vi "Aurora Reader (Dual Port).vi"(2 "aurora rx dual reference":T1, 12 "ready for output":bool=TRUE) -> (4 "data":bool[](array[boolean]), 10 "output valid":bool)   [LabVIEW 2019]
uses:
  <vilib>/eio/EIONode/EIONode.xnode
  <instrlib>/_niInstr/Data Formatting/v1/FPGA/niInstr Data Formatting v1 FPGA.lvlib
  <instrlib>/_niInstr/Data Formatting/v1/FPGA/Private/Convert/U64 array to Boolean Array.vi
  <vilib>/rvi/eio/common/nirviEmuTemplateMethod_errors.vi
  Aurora RX Dual Reference.ctl
  AXI4-Stream Reader FXP64x4 Resources.ctl
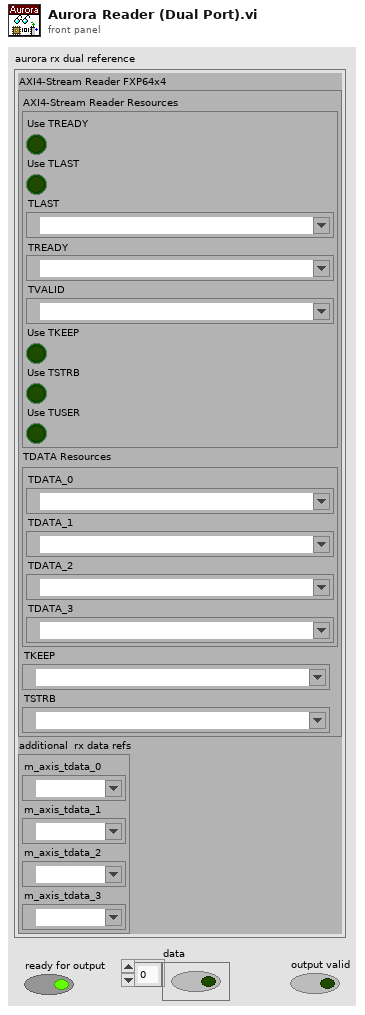
[diagram p1: front panel]
types:
  T1 = typedef "Aurora RX Dual Reference.ctl" = cluster{"AXI4-Stream Reader FXP64x4":T2, "additional  rx data refs":cluster{"m_axis_tdata_0":refnum<k21>, "m_axis_tdata_1":refnum<k21>, "m_axis_tdata_2":refnum<k21>, "m_axis_tdata_3":refnum<k21>}}
  T2 = typedef "AXI4-Stream Reader FXP64x4 Resources.ctl" = cluster{"AXI4-Stream Reader Resources":cluster{"Use TREADY":bool, "Use TLAST":bool, "TLAST":refnum<k21>, "TREADY":refnum<k21>, "TVALID":refnum<k21>, "Use TKEEP":bool, "Use TSTRB":bool, "Use TUSER":bool}, "TDATA Resources":cluster{"TDATA_0":refnum<k21>, "TDATA_1":refnum<k21>, "TDATA_2":refnum<k21>, "TDATA_3":refnum<k21>}, "TKEEP":refnum<k21>, "TSTRB":refnum<k21>}
  T3 = cluster{"m_axis_tdata_0":refnum<k21>, "m_axis_tdata_1":refnum<k21>, "m_axis_tdata_2":refnum<k21>, "m_axis_tdata_3":refnum<k21>}
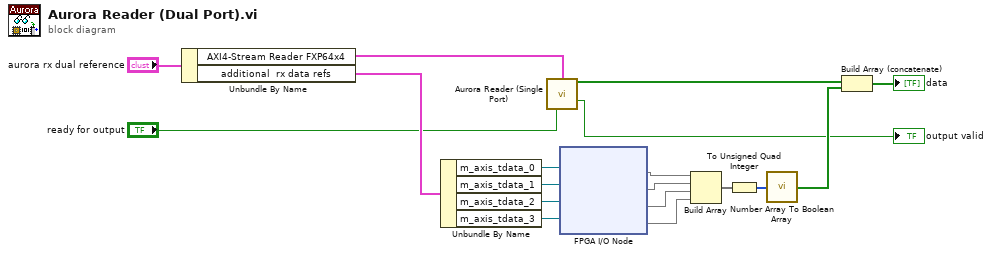
[diagram p0: block diagram]
diagram:
  n1 = Unbundle By Name("aurora rx dual reference") -> ("AXI4-Stream Reader FXP64x4"=w1:T2, "additional  rx data refs"=w18:T3)
  n2 = Unbundle By Name(w18) -> ("m_axis_tdata_0"=w17:refnum<k21>, "m_axis_tdata_1"=w16:refnum<k21>, "m_axis_tdata_2"=w15:refnum<k21>, "m_axis_tdata_3"=w14:refnum<k21>)
  n3 = call "Aurora Reader (Single Port) .vi"("AXI4-Stream Reader FXP64x4"=w1, "ready for output"="ready for output") -> ("data"=w2:bool[], "output valid"=→"output valid":bool)  [unwired: 12 in]
  n4 = xnode "FPGA I/O Node"("FPGA I/O In"=w17, "FPGA I/O In"=w16, "FPGA I/O In"=w15, "FPGA I/O In"=w14) -> ("I/O Item"=w11, "I/O Item"=w10, "I/O Item"=w9, "I/O Item"=w8)  [unwired: 4 out]
  n5 = Build Array(w11, w10, w9, w8) -> (w13:void[])
  n6 = To Unsigned Quad Integer(1:w13) -> (0:w12:u64[])
  n7 = call-poly <instrlib>:"Number Array To Boolean Array.vi"("data in"=w12) -> ("data out"=w7:bool[])  [unwired: 14 in]
  n8 = Build Array (concatenate)(w2, w7) -> (→"data":bool[])
